vi "ShowSampleInfo.vi"(8 "error in (no error)":errorcluster, 10 "Analysis in":refnum<class "Analysis.lvclass">, 11 "Table Control":refnum<vi>) -> (0 "error out":errorcluster)   [LabVIEW 2015]
doc: "Loads the SampleInfo from the AnalysisObject and displays the data in the Table"
uses:
  MSControl/Classes/Analysis/Analysis.lvclass
  <vilib>/Utility/miscctls.llb/LVRowAndColumnUnsignedTypeDef.ctl
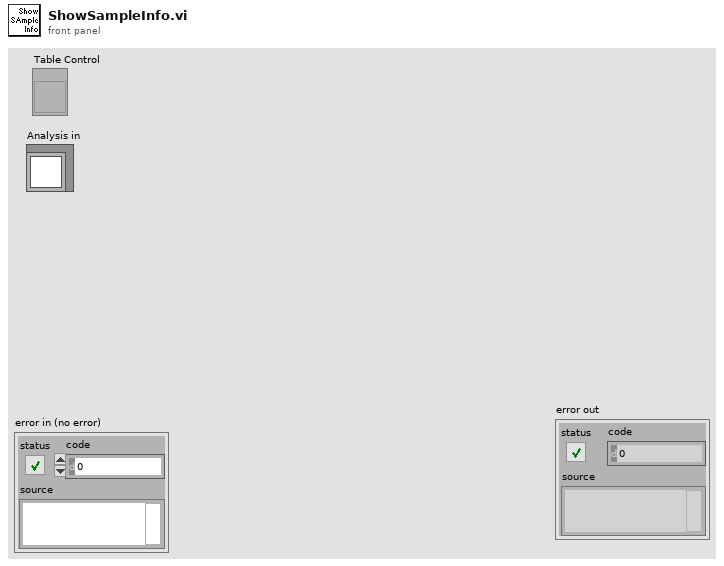
[diagram p1: front panel]
types:
  T1 = typedef "LVRowAndColumnUnsignedTypeDef.ctl" = cluster{"Row":u32, "Column":u32}
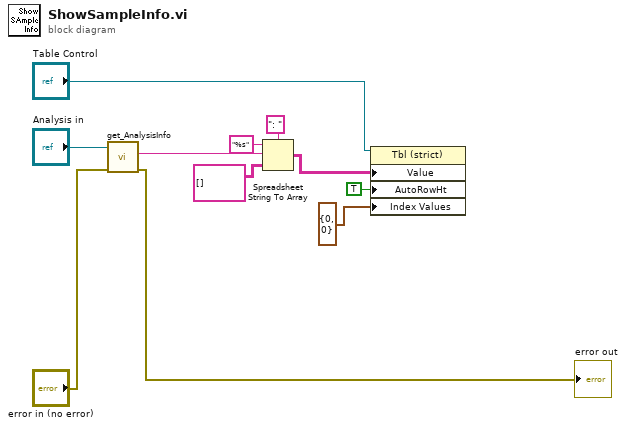
[diagram p0: block diagram]
diagram:
  n1 = call "get_AnalysisInfo.vi"("error in (no error)"="error in (no error)", "Analysis in"="Analysis in") -> ("error out"=→"error out":errorcluster, "AnalysisInfo out"=w8:string)  [unwired: 7 in, 1 out]
  n2 = Spreadsheet String To Array(delimiter (Tab)=": ", format string="%s", spreadsheet string=w8, array type (2D Dbl)=string[][] []) -> (array=w3:string[][])
  n3 = property class="Tbl (strict)"(reference="Table Control", "Value"=w3, "AutoRowHt"=TRUE ("Autosizing Row Height"), "Index Values"=T1 {"Row"=0, "Column"=0}) -> ()  [unwired: 1 in, 2 out]
